vi "Easy Gabor Transform.vi"(8 "error in (no error)":errorcluster, 9 "window info":T1={"window type"=10, "window length"=2048} {"window type" items=["None"=0, "Hanning"=1, "Hamming"=2, "Blackman-Harris"=3, "Exact Blackman"=4, "Blackman"=5, "Flat Top"=6, "4 Term B-Harris"=7, "7 Term B-Harris"=8, "Low Sidelobe"=9, "Gaussian"=62]; "window length" min=0}, 10 "x[n]":dbl[](array[numeric]) format="%.2f", 11 "RefNum in":T2) -> (0 "error out":errorcluster, 1 "actual window":T1={"window type"=10, "window length"=2048} {"window type" items=["None"=0, "Hanning"=1, "Hamming"=2, "Blackman-Harris"=3, "Exact Blackman"=4, "Blackman"=5, "Flat Top"=6, "4 Term B-Harris"=7, "7 Term B-Harris"=8, "Low Sidelobe"=9, "Gaussian"=62]; "window length" min=0}, 3 "RefNum out":T2, 4 "synthesis window":cluster{"g[i]":dbl[], "dM":i32, "length":i32} {"g[i]" format="%.2f"}, 5 "analysis window":cluster{"gamma[i]":dbl[], "dM":i32, "N":i32} {"gamma[i]" format="%.2f"})   [LabVIEW 2017, in "SoundVib_Gabor.lvlib"]
doc: "Performs a Gabor transform on <B>x[n]</B>. The VI stores the resulting Gabor coefficients in the data block referenced by <B>RefNum in</B>. You can retrieve the stored coefficients with the Get Gabor Coefficients VI."
uses:
  <vilib>/addons/Sound and Vibration/Order Analysis/Gabor Order Tracking/SoundVib_Gabor.lvlib
  <vilib>/addons/Sound and Vibration/Order Analysis/Ref Gabor Order Tracking/GT RefNum.ctl
  <vilib>/addons/Sound and Vibration/Order Analysis/Ref Gabor Order Tracking/window information.ctl
  <resource>/sndvib.dll
panel:
  # "Easy Gabor Transform"
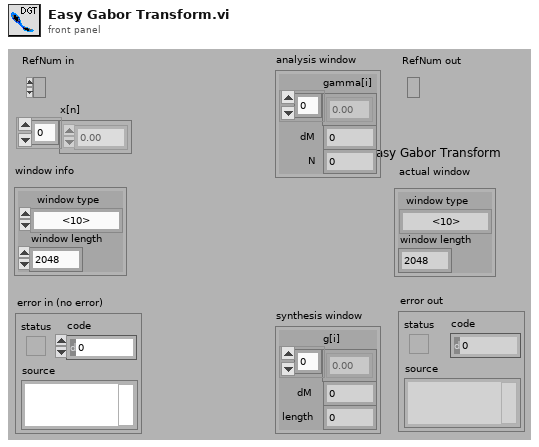
[diagram p1: front panel]
types:
  T1 = typedef "SoundVib_Gabor.lvlib/window information.ctl" = cluster{"window type":u32, "window length":i32}
  T2 = typedef "SoundVib_Gabor.lvlib/GT RefNum.ctl" = refnum<k1>
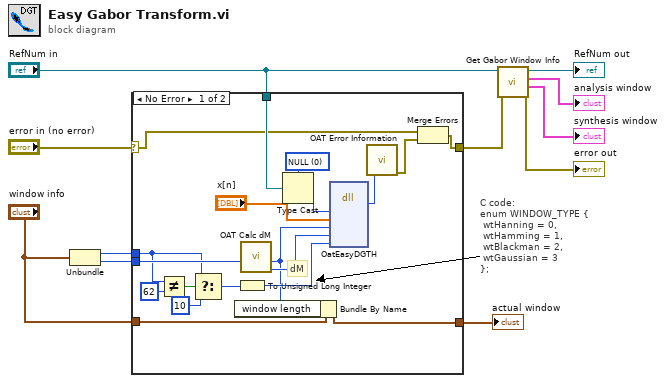
[diagram p0: block diagram]
diagram:
  # "C code:\nenum WINDOW_TYPE {\n\twtHanning = 0,\n\twtHamming = 1,\n\twtBlackman = 2,\n\twtGaussian = 3\n};"
  n1 = Unbundle("window info") -> ("window type"=w3:u32, "window length"=w4:i32)
  n2 = case shown="No Error" "error in (no error)" {
    selector: "error in (no error)" -> [w14 w32]
    tunnel: [w12 w32] -> w8
    tunnel: w4 -> [w25 _]
    tunnel: "RefNum in" -> [w23 _]
    tunnel: w3 -> [w17 _]
    tunnel: "window info" -> [w22 w31]
    tunnel: [w20 w31] -> w9
    frame No Error {
      w27 = u32 0 items=["NULL"]
      # "dM"
      n3 = Not Equal?(x=w17, y=u32 62) -> (x != y?=w18:bool)
      n4 = Select(t=w17, s=w18, f=u32 10) -> (s? t:f=w15:u32)
      n5 = To Unsigned Long Integer(number=w15) -> (unsigned 32bit integer=w29:u32)
      n6 = call <vilib>:"OAT Calc dM.vi"("window length"=w25) -> ("dM"=w24:i32, "actual window length"=w21:i32)  [unwired: 7 in, 2 out]
      n7 = Bundle By Name(cluster=w22, "window length"=w21) -> (w20:T1)
      n8 = Type Cast(type=w27, x=w23) -> (*(type *) &x=w28:u32)
      n9 = dll-call lib="C:/Program Files (x86)/National Instruments/LabVIEW 2017/resource/sndvib.*" fn="OatEasyDGTH"("Ref In"=w28, "InputArray"="x[n]", "WindowLength"=w21, "dM"=w24, "Window Type"=w29) -> ("return type"=w26:i32)  [unwired: 8 in, 2 out]
      n10 = call <vilib>:"OAT Error Information.vi"("error code"=w26) -> ("error out"=w13:errorcluster)  [unwired: 6 in]
      n11 = Merge Errors(w14, w13) -> (w12:errorcluster)
    }
    frame Error {
    }
  }
  "actual window" <- w9
  n12 = call <vilib>:"Get Gabor Window Info.vi"("error in (no error)"=w8, "RefNum in"="RefNum in") -> ("error out"=→"error out":errorcluster, "synthesis window"=→"synthesis window":cluster{"g[i]":dbl[], "dM":i32, "length":i32}, "analysis window"=→"analysis window":cluster{"gamma[i]":dbl[], "dM":i32, "N":i32}, "RefNum out"=→"RefNum out":T2)  [unwired: 6 in]
